vi "ECG QRS Complex Detection.vi"() -> ()   [LabVIEW 2023]
doc: "This example shows the application of wavelet-based peak detection in biomedical engineering.\n\nThe peaks in an electrocardiogram (ECG) signal indicate the rhythm of the heart, which is one of the key characteristics of the human body. Typically one lead of an ECG signal consists of five peaks and valleys. The first positive deflection is referred to as the P wave. The following negative deflection is the Q wave. The following positive deflection after the Q wave is the R wave. The negative deflection after the R wave is the S wave. The following positive deflection after the S wave is the T wave. The duration between the Q and S waves is called the QRS duration. The QRS duration indicates the ventricular condition. The peaks in ECG signals usually are corrupted by environment noise and cannot be detected properly by traditional curving-fitting methods. The wavelet-based peak detection method is naturally immune to noise and can detect both sharp and mild peaks/valleys accurately. The wavelet-based method also is less affected by the trend in the signal. \n\nThis example uses the WA Multiscale Peak Detection VI to detect the peaks in an ECG signal and computes the QRS duration.\n\n<b>Instructions:</b>\n1) Run this VI.\n2) Change the value of the <b>Peak/Valley Width</b> and observe the peak detection results."
uses:
  <vilib>/addons/Wavelet Analysis/typedefs.llb/WA Data.ctl
  <vilib>/addons/Wavelet Analysis/online wavelet analysis.llb/WA Online Multiscale Peak Detection (Array).vi
  <vilib>/addons/_Advanced Signal Processing/NI_AdvSigProcWA.lvlib
  <vilib>/addons/_Advanced Signal Processing/NI_AdvSigProcOnlineWA.lvlib
panel:
  out "aspt-left-top":bool
  in  "stop":bool
  out "QRS Duration":dbl[](graph)
  out "Peaks/Valleys Plot":cluster{"Ramp Pattern":dbl[], "X":dbl[]}[](graph)
  in  "Peak/Valley width":i32=32
  # "Overview: Shows the application of wavelet-based peak detection in biomedical engineering.\nRequirements: LabVIEW Full Development System, Advanced Signal Processing Toolkit\nInstructions: \n1. Run this VI.\n2. Change the value of the Peak/Valley Width and observe the peak detection results.\n3. Click Stop to stop the VI."
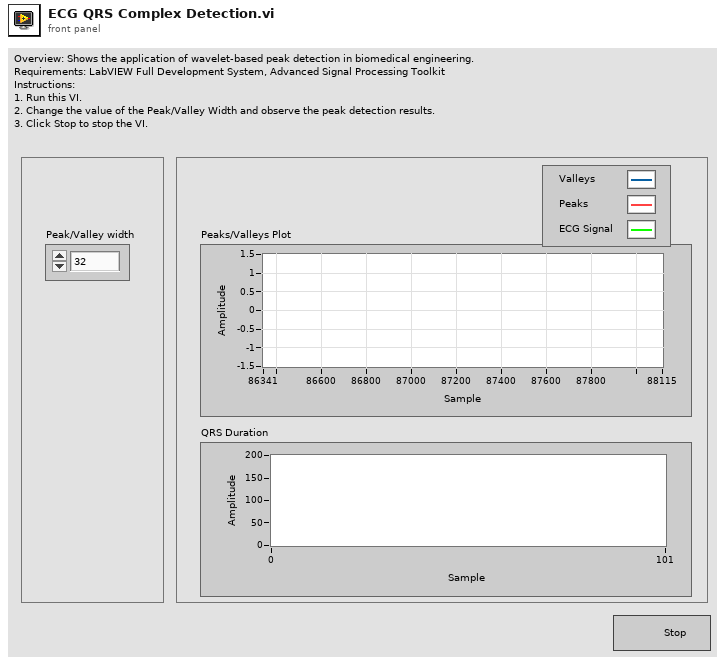
[diagram p1: front panel]
types:
  T1 = typedef "NI_AdvSigProcWA.lvlib/WA Data.ctl" = u16
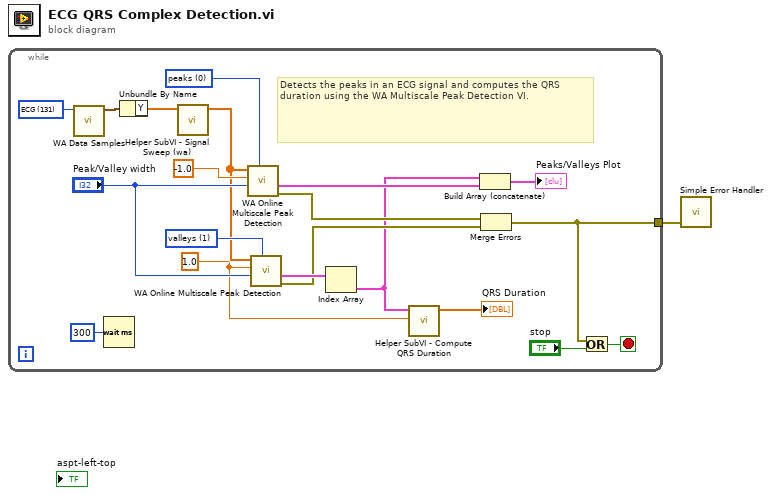
[diagram p0: block diagram]
diagram:
  n1 = while {
    tunnel: [w2] -> w1
    stop <- w19 stop-if-true
    w6 = T1 131 items=["1D Example Data"=100, "-"=101, "Doppler"=102, "HOP"=103, "TF Sine"=104, "Noisy Doppler"=105, "Sea Temperature"=106, "Sp500"=107, "Power Line"=108, "Engine Knocking"=109, "HeaviSine"=110, "Bumps"=111, "Blocks"=112, "Piece Regular"=113, "HypChirps"=114, "LinChirps"=115, "Chirps"=116, "Piece Polynomial"=117, "ECG"=131, "-"=118, "2D Example Data"=119, "-"=120, "Finger Print (Image)"=121, "Iris Flower (Image)"=122, "Mammogram (Image)"=123, "Lake (Image)"=127, "Two Can 1 (Image)"=132, "Two Can 2 (Image)"=133, "Camera Man (Image)"=134] ("data")
    w3 = 1.0 ("threshold")
    w14 = u16 0 items=["peaks", "valleys"] ("peaks/valleys")
    w13 = u16 1 items=["peaks", "valleys"] ("peaks/valleys")
    # "Detects the peaks in an ECG signal and computes the QRS duration using the WA Multiscale Peak Detection VI."
    n2 = call <vilib>:"WA Data Samples.vi"("data"=w6) -> ("signal"=w17:waveform(dbl))  [unwired: 10 out]
    n3 = Wait (ms)(milliseconds to wait=u32 300 ("millisecond multiple")) -> ()  [unwired: 1 out]
    n4 = Unbundle By Name(w17) -> ("Y"=w16:dbl[])
    n5 = call "Helper SubVI - Signal Sweep (wa).vi"("Signal in"=w16) -> ("Signal out"=w5:dbl[])  [unwired: 10 in]
    n6 = call-poly <vilib>:"WA Online Multiscale Peak Detection.vi"("peaks/valleys"=w14, "width"="Peak/Valley width", "threshold"=-1.0 ("Threshold"), "signal"=w5) -> ("error out"=w10:errorcluster, "peak plot"=w21:cluster{"Ramp Pattern":dbl[], "X":dbl[]}[])  [unwired: 4 in, 2 out]
    n7 = call-poly <vilib>:"WA Online Multiscale Peak Detection.vi"("peaks/valleys"=w13, "width"="Peak/Valley width", "threshold"=w3, "signal"=w5) -> ("error out"=w9:errorcluster, "peak plot"=w12:cluster{"Ramp Pattern":dbl[], "X":dbl[]}[])  [unwired: 4 in, 2 out]
    n8 = Index Array(array=w12) -> (element=w7:cluster{"Ramp Pattern":dbl[], "X":dbl[]})  [unwired: 1 in]
    n9 = call "Helper SubVI - Compute QRS Duration.vi"("threshold"=w3, "valleys"=w7) -> ("QRS Duration"=→"QRS Duration":dbl[])  [unwired: 9 in]
    n10 = Build Array (concatenate)(w7, w21) -> (→"Peaks/Valleys Plot":cluster{"Ramp Pattern":dbl[], "X":dbl[]}[])
    n11 = Merge Errors(w10, w9) -> (w2:errorcluster)
    n12 = Or(x=w2, y="stop") -> (x .or. y?=w19:bool)
  }
  n13 = call <vilib>:"Simple Error Handler.vi"("error in (no error)"=w1) -> ()  [unwired: 1 in, 8 out]
